vi "Error Complete Call Chain.vi"(8 "error in (no error)":errorcluster) -> (0 "error out":errorcluster)   [LabVIEW 2013, in "Utilities 1.lvlib"]
uses:
  Utilities 1.lvlib
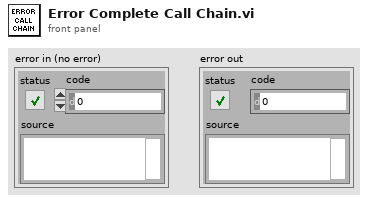
[diagram p1: front panel]
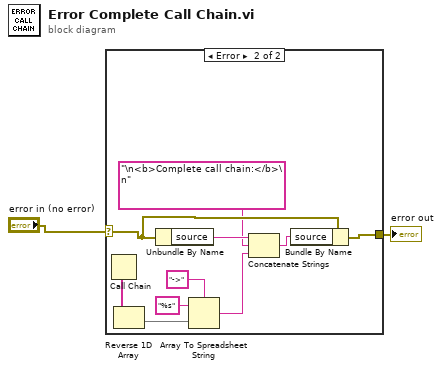
[diagram p0: block diagram]
diagram:
  n1 = case shown="Error" "error in (no error)" {
    selector: "error in (no error)" -> [w3 w13]
    tunnel: [w3 w10] -> w2
    frame No Error {
    }
    frame Error {
      n2 = Call Chain() -> (call chain=w8:string[])
      n3 = Reverse 1D Array(array=w8) -> (reversed array=w6:string[])
      n4 = Unbundle By Name(w13) -> ("source"=w12:string)
      n5 = Array To Spreadsheet String(delimiter (Tab)="->", array=w6, 3:"%s" ("format string")) -> (spreadsheet string=w4:string)
      n6 = Concatenate Strings(w12, "\n<b>Complete call chain:</b>\n" ("search string/char (-)"), w4) -> (w11:string)
      n7 = Bundle By Name(cluster=w13, "source"=w11) -> (w10:errorcluster)
    }
  }
  "error out" <- w2
